vi "toStringArray.vi"(8 "error in (no error)":errorcluster, 11 "RampToneAmplitudeDown in":refnum<class "RampToneAmplitudeDown.lvclass">) -> (0 "error out":errorcluster, 2 "eventStringArray":string[](array[string]), 3 "RampToneAmplitudeDown out":refnum<class "RampToneAmplitudeDown.lvclass">)   [LabVIEW 2011, in "Tools.lvlib" / "Scripting.lvlib" / "RampToneAmplitudeDown.lvclass"]
uses:
  RampToneAmplitudeDown.lvclass
  RampTone/RampTone.lvclass
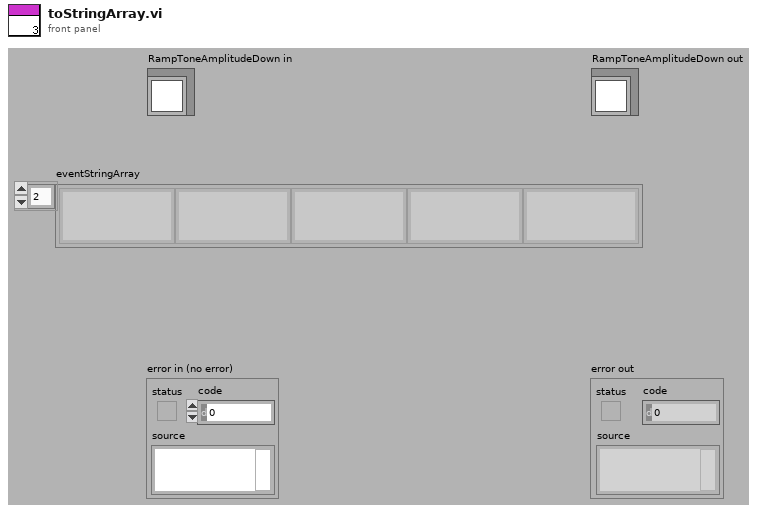
[diagram p1: front panel]
types:
  T1 = cluster{"rampTime":dbl, "timeStep":dbl, "dataValueStep":dbl}
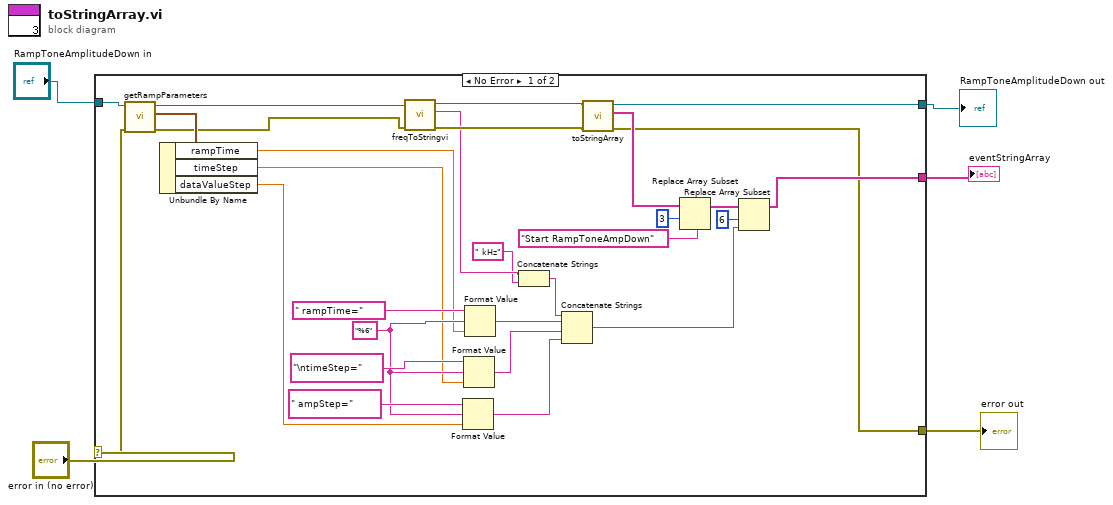
[diagram p0: block diagram]
diagram:
  n1 = case shown="No Error" "error in (no error)" {
    selector: "error in (no error)" -> [w6 w35]
    tunnel: [w17 w35] -> w1
    tunnel: [w24 _] -> w2
    tunnel: "RampToneAmplitudeDown in" -> [w13 w36]
    tunnel: [w20 w36] -> w3
    frame No Error {
      w23 = "%6"
      n2 = call "getRampParameters.vi"("error in (no error)"=w6, "RampTone in"=w13) -> ("error out"=w7:errorcluster, "RampParameters"=w11:T1, "RampTone out"=w12:refnum<class "RampToneAmplitudeDown.lvclass">)  [unwired: 7 in]
      n3 = Unbundle By Name(w11) -> ("rampTime"=w10:dbl, "timeStep"=w9:dbl, "dataValueStep"=w8:dbl)
      n4 = call-dynamic "freqToStringvi.vi"("error in (no error)"=w7, "SingleTone in"=w12) -> ("error out"=w18:errorcluster, "frequency"=w15:string, "SingleTone out"=w21:refnum<class "RampToneAmplitudeDown.lvclass">)  [unwired: 7 in]
      n5 = Format Value(string ("")=" ampStep=", format string=w23, value (0)=w8) -> (output string=w16:string)
      n6 = Format Value(string ("")="\ntimeStep=", format string=w23, value (0)=w9) -> (output string=w26:string)
      n7 = Format Value(string ("")=" rampTime=", format string=w23, value (0)=w10) -> (output string=w27:string)
      n8 = Concatenate Strings(w15, " kHz") -> (w22:string)
      n9 = Concatenate Strings(w22, w27, w26, w16) -> (w25:string)
      n10 = call-parent "toStringArray.vi"("error in (no error)"=w18, "RampTone in"=w21) -> ("error out"=w17:errorcluster, "eventStringArray"=w19:string[], "RampTone out"=w20:refnum<class "RampToneAmplitudeDown.lvclass">)  [unwired: 7 in]
      n11 = Replace Array Subset(array=w19, new element="Start RampToneAmpDown", index=3) -> (w30:string[])
      n12 = Replace Array Subset(array=w30, new element=w25, index=6) -> (w24:string[])
    }
    frame Error {
    }
  }
  "error out" <- w1
  "RampToneAmplitudeDown out" <- w3
  "eventStringArray" <- w2
